vi "Begin.vi"(11 "Image Size":T1=enum."160x120") -> (0 "error out":errorcluster)   [LabVIEW 2011]
doc: "Called before other user functions, this VI is expected to open initial I/O refnums, load in file data, and do all program initialization. Notice that the <B>error out</B> terminal is simply used for data flow. Wiring it to other structures or subVIs ensures that this VI runs first."
uses:
  <vilib>/Rock Robotics/WPI/Camera/WPI_CameraImageSize.ctl
  <vilib>/Rock Robotics/WPI/Joystick/WPI_JoystickDeviceEnum.ctl
  <vilib>/Rock Robotics/WPI/Camera/WPI_CameraWhite Balance Values.ctl
  <vilib>/Rock Robotics/WPI/Camera/WPI_CameraExposure Values.ctl
  <vilib>/Rock Robotics/WPI/Camera/WPI_CameraFrameRate.ctl
  <vilib>/Rock Robotics/SystemInterfaces/DIO/FPGA_DIOPWMChannel.ctl
  <vilib>/Rock Robotics/SystemInterfaces/DIO/FPGA_DIOChannel.ctl
  <vilib>/Rock Robotics/SystemInterfaces/DIO/FPGA_DIORelayChannel.ctl
  <vilib>/Rock Robotics/WPI/RobotDrive/WPI_RobotDriveOpen4MotorWithJaguar.vi
  <vilib>/Rock Robotics/WPI/MotorControl/WPI_MotorControlOpen Jaguar.vi
  <vilib>/Rock Robotics/WPI/Counter/WPI_CounterDigitalInputToDigitalSource.vi
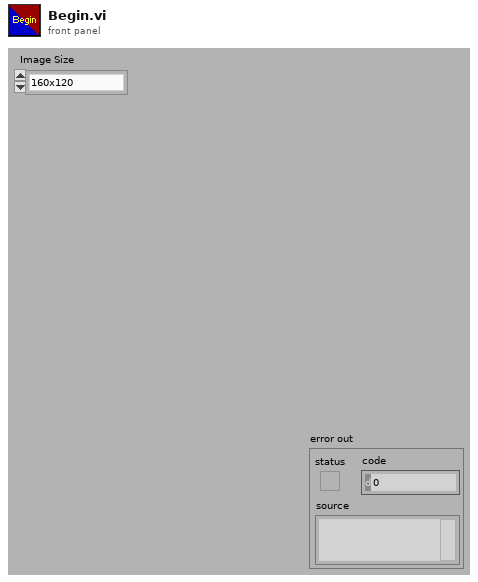
[diagram p1: front panel]
types:
  T1 = typedef "WPI_CameraImageSize.ctl" = enum16{"640x480", "320x240", "160x120"}
  T2 = typedef "FPGA_DIORelayChannel.ctl" = enum8{"Relay 1", "Relay 2", "Relay 3", "Relay 4", "Relay 5", "Relay 6", "Relay 7", "Relay 8", "Invalid"}
  T3 = typedef "FPGA_DIOChannel.ctl" = enum8{"DIO 1", "DIO 2", "DIO 3", "DIO 4", "DIO 5", "DIO 6", "DIO 7", "DIO 8", "DIO 9", "DIO 10", "DIO 11", "DIO 12", "DIO 13", "DIO 14", "Invalid"}
  T4 = typedef "FPGA_DIOPWMChannel.ctl" = enum8{"PWM 1", "PWM 2", "PWM 3", "PWM 4", "PWM 5", "PWM 6", "PWM 7", "PWM 8", "PWM 9", "PWM 10", "Invalid"}
  T5 = typedef "WPI_JoystickDeviceEnum.ctl" = enum16{"USB 1", "USB 2", "USB 3", "USB 4", "Kinect 1", "Kinect 2"}
  T6 = typedef "WPI_CameraFrameRate.ctl" = u32
  T7 = typedef "WPI_CameraExposure Values.ctl" = enum16{"Auto", "Flicker-free 50 Hz", "Flicker-free 60 Hz", "Hold current"}
  T8 = typedef "WPI_CameraWhite Balance Values.ctl" = enum16{"Auto", "Fixed indoor", "Fixed outdoor 1", "Fixed outdoor 2", "Fixed fluorescent 1", "Fixed fluorescent 2", "Hold current"}
  T9 = typedef "WPI_DigitalInputDevRef.ctl" = cluster{"DevStatus":errorcluster, "DIO Channel":T3, "Digital Module":T10}
  T10 = typedef "FPGA_TypedefDigitalModule.ctl" = enum16{"Digital Module 1", "Digital Module 2"}
  T11 = typedef "FPGA_CounterEncoderSourceConvertionLVSourceType.ctl" = cluster{"DevStatus":errorcluster, "AnalogTriggerMode?":bool, "DigitalMode":cluster{"Digital Module":T10, "DIO Channel":T12}, "AnalogTriggerMode":cluster{"AnalogTriggerIndex":T13, "OutputType":T14}}
  T12 = typedef "FPGA_DIODigitalSourceChannel.ctl" = enum8{"DIO 1", "DIO 2", "DIO 3", "DIO 4", "DIO 5", "DIO 6", "DIO 7", "DIO 8", "DIO 9", "DIO 10", "DIO 11", "DIO 12", "DIO 13", "DIO 14", "Disabled"}
  T13 = typedef "FPGA_AnalogTriggerIndex.ctl" = enum8{"Trig 0", "Trig 1", "Trig 2", "Trig 3", "Trig 4", "Trig 5", "Trig 6", "Trig 7", "Invalid"}
  T14 = typedef "FPGA_AnalogTriggerOutType.ctl" = enum16{"InWindow", "TriggerState", "Rising", "Falling"}
  T15 = typedef "WPI_EncoderDevRef.ctl" = cluster{"DevStatus":errorcluster, "EncoderIndex":T16, "CounterIndex":T17, "DistancePerCount":dbl, "Decoding Type":T18}
  T16 = typedef "FPGA_EncoderIdx.ctl" = enum8{"Enc 0", "Enc 1", "Enc 2", "Enc 3", "Invalid"}
  T17 = typedef "FPGA_CounterCtrSystemIndex.ctl" = enum8{"Ctr 0", "Ctr 1", "Ctr 2", "Ctr 3", "Ctr 4", "Ctr 5", "Ctr 6", "Ctr 7", "Invalid"}
  T18 = typedef "WPI_EncoderType.ctl" = enum16{"1x", "2x", "4x"}
  T19 = typedef "WPI_JoystickDevRef.ctl" = cluster{"Device":T5}
  T20 = typedef "WPI_MotorControlDeviceRef.ctl" = cluster{"DeviceStatus":errorcluster, "Type":enum16{"PWM", "CAN"}, "PWM":cluster{"Digital Module":T10, "PWM Channel":T4, "DeadBand":T21}, "CAN":cluster{"Device Number":u8, "Control Mode":T22, "Semaphore":T23, "Max Vout":dbl}, "Invert":bool, "TransformRef":T24, "InvTransformRef":T24}
  T21 = typedef "WPI_PWMDeadband.ctl" = cluster{"Name":string, "maxPositivePwm":i32, "minPositivePwm":i32, "centerPwm":i32, "maxNegativePwm":i32, "minNegativePwm":i32, "angularRange":u16}
  T22 = typedef "WPI_CANJaguar_ControlMode.ctl" = enum8{"Percent VBus", "Current", "Speed", "Position", "Voltage"}
  T23 = typedef "Semaphore RefNum" = refnum<k1>
  T24 = typedef "WPI_PWMTransform_ConPane.ctl" = refnum<vi>
  T25 = typedef "WPI_RobotDriveDevRef.ctl" = cluster{"DevStatus":errorcluster, "Motors[]":T20[], "Square Inputs":bool, "Max Output":dbl, "Isochronous":bool}
  T26 = typedef "WPI_CameraDevRef.ctl" = cluster{"Camera Address":string, "CameraStatus":errorcluster, "Acquire Image Notifier":refnum<notifier>}
  T27 = typedef "WPI_RelayDevRef.ctl" = cluster{"DevStatus":errorcluster, "Relay Channel":T2, "Digital Module":T10, "Relay Direction":T28}
  T28 = typedef "WPI_RelayDirection.ctl" = enum16{"Both directions", "Forward only", "Reverse only"}
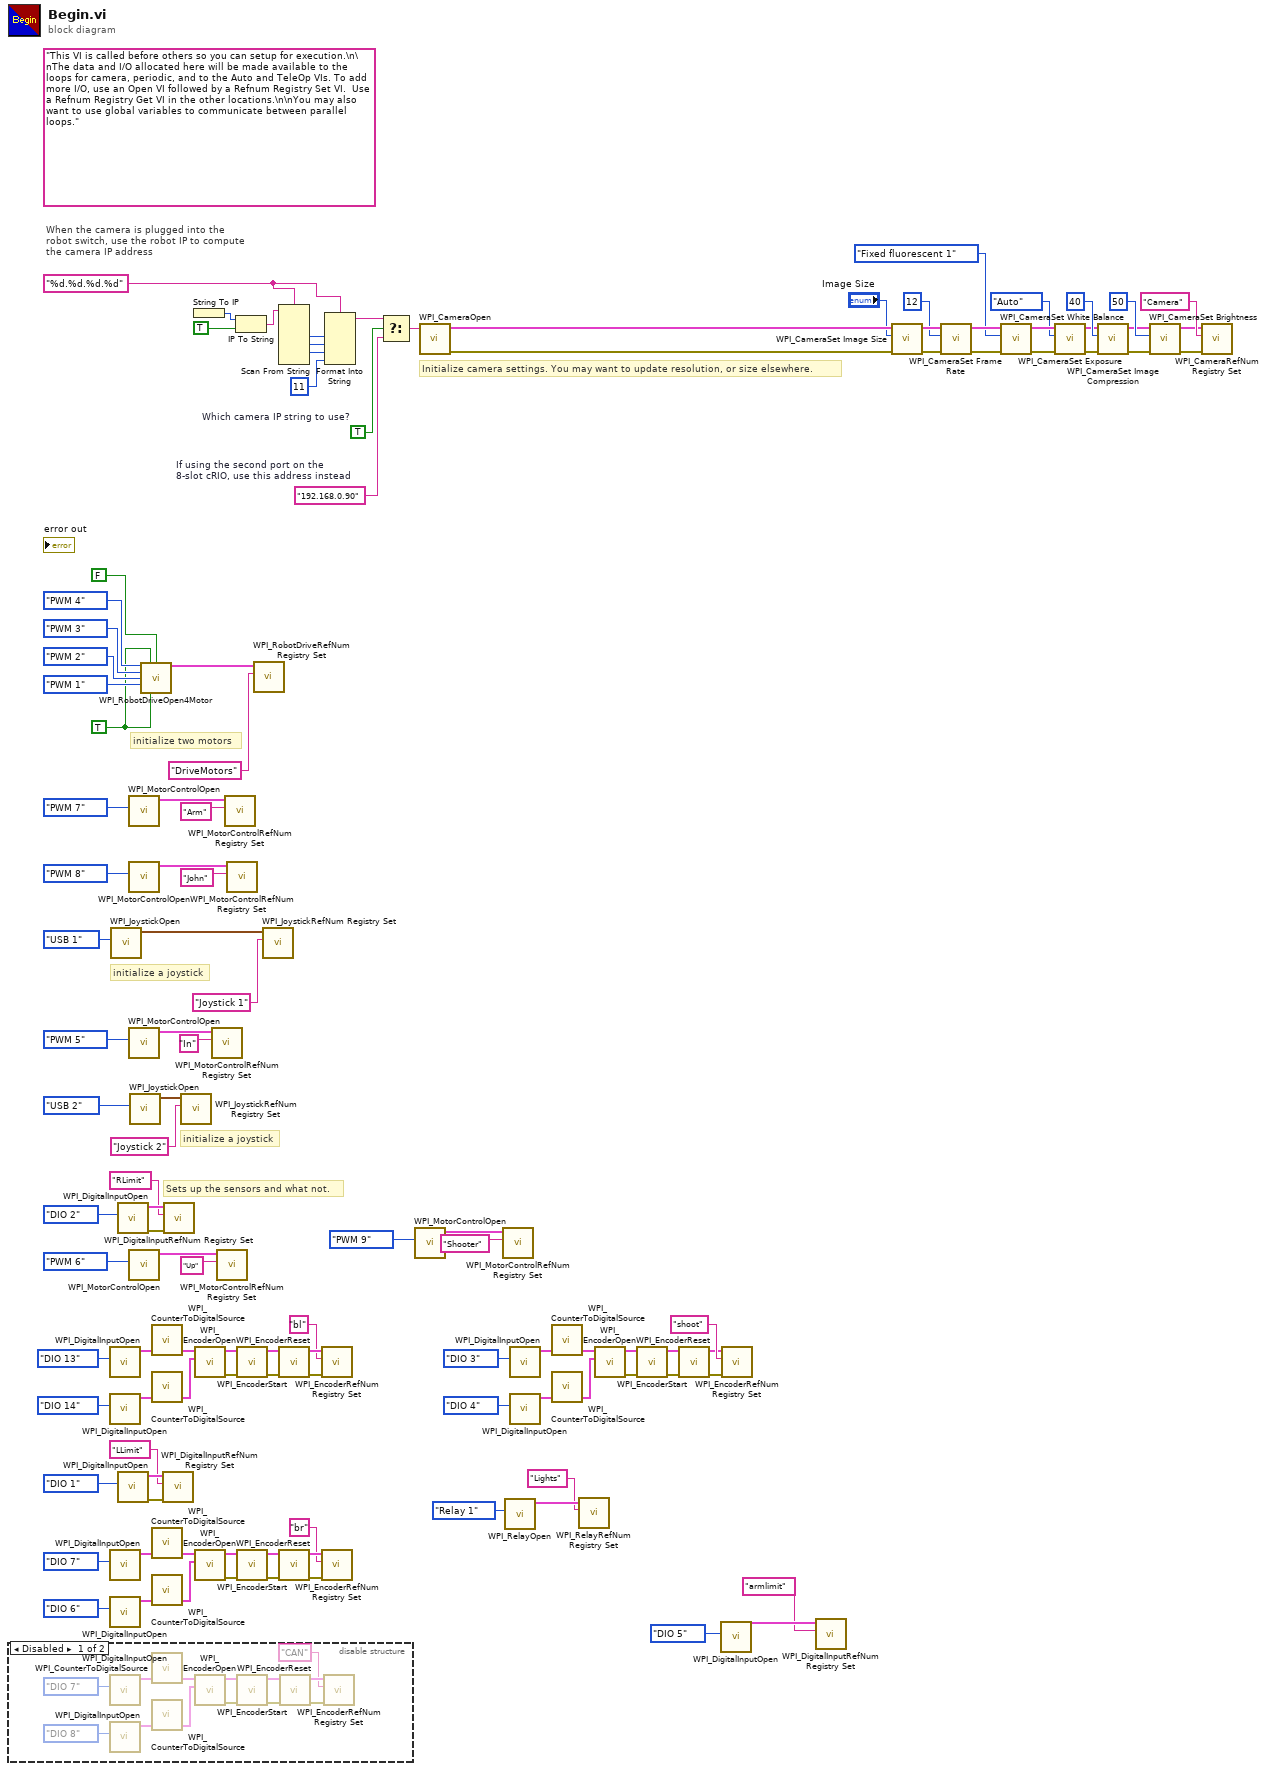
[diagram p0: block diagram]
diagram:
  w49 = TRUE ("Rear Left Motor Inverted")
  w79 = TRUE  # Which camera IP string to use?
  w83 = "%d.%d.%d.%d" ("format string")
  (unwired) "This VI is called before others so you can setup for execution.\n\nThe data and I/O allocated here will be made available to the loops for camera, periodic, and to the Auto and TeleOp VIs. To add more I/O, use an Open VI followed by a Refnum Registry Set VI.  Use a Refnum Registry Get VI in the other locations.\n\nYou may also want to use global variables to communicate between parallel loops."
  w80 = "192.168.0.90"  # If using the second port on the 8-slot cRIO, use this address instead
  # "Sets up the sensors and what not."
  # "initialize a joystick"
  # "When the camera is plugged into the\nrobot switch, use the robot IP to compute\nthe camera IP address"
  # "initialize a joystick"
  # "initialize two motors"
  # "Initialize camera settings. You may want to update resolution, or size elsewhere."
  n1 = disable-structure shown="Disabled" {
    frame Disabled {
      n2 = call <vilib>:"WPI_DigitalInputOpen.vi"("DIO Channel"=FPGA_DIOChannel."DIO 7") -> ("DigitalInputDevRef"=w126:T9)  [unwired: 9 in, 1 out]
      n3 = call <vilib>:"WPI_DigitalInputOpen.vi"("DIO Channel"=FPGA_DIOChannel."DIO 8") -> ("DigitalInputDevRef"=w125:T9)  [unwired: 9 in, 1 out]
      n4 = call-poly <vilib>:"WPI_CounterToDigitalSource.vi"("DigitalInputDevRef"=w126) -> ("Digital Source"=w128:T11)  [unwired: 6 in]
      n5 = call-poly <vilib>:"WPI_CounterToDigitalSource.vi"("DigitalInputDevRef"=w125) -> ("Digital Source"=w127:T11)  [unwired: 6 in]
      n6 = call <vilib>:"WPI_EncoderOpen.vi"("BSource"=w127, "ASource"=w128) -> ("error out"=w122:errorcluster, "EncoderDevRef"=w121:T15)  [unwired: 8 in]
      n7 = call <vilib>:"WPI_EncoderStart.vi"("error in (no error)"=w122, "EncoderDevRef"=w121) -> ("error out"=w120:errorcluster, "EncoderDevRef"=w119:T15)  [unwired: 8 in]
      n8 = call <vilib>:"WPI_EncoderReset.vi"("error in (no error)"=w120, "EncoderDevRef"=w119) -> ("error out"=w118:errorcluster, "EncoderDevRef"=w117:T15)  [unwired: 8 in]
      n9 = call <vilib>:"WPI_EncoderRefNum Registry Set.vi"("error in (no error)"=w118, "refnum name"="CAN", "EncoderDevRef"=w117) -> ()  [unwired: 7 in, 2 out]
    }
    frame Enabled {
    }
  }
  n10 = call <vilib>:"WPI_DigitalInputOpen.vi"("DIO Channel"=FPGA_DIOChannel."DIO 13") -> ("DigitalInputDevRef"=w48:T9)  [unwired: 9 in, 1 out]
  n11 = call <vilib>:"WPI_DigitalInputOpen.vi"("DIO Channel"=FPGA_DIOChannel."DIO 14") -> ("DigitalInputDevRef"=w43:T9)  [unwired: 9 in, 1 out]
  n12 = call <vilib>:"WPI_DigitalInputOpen.vi"("DIO Channel"=FPGA_DIOChannel."DIO 7") -> ("DigitalInputDevRef"=w42:T9)  [unwired: 9 in, 1 out]
  n13 = call <vilib>:"WPI_DigitalInputOpen.vi"("DIO Channel"=FPGA_DIOChannel."DIO 6") -> ("DigitalInputDevRef"=w41:T9)  [unwired: 9 in, 1 out]
  n14 = call <vilib>:"WPI_JoystickOpen.vi"("JoystickDevice"=WPI_JoystickDeviceEnum."USB 1") -> ("JoystickDevRef"=w113:T19)  [unwired: 10 out]
  n15 = call <vilib>:"WPI_DigitalInputOpen.vi"("DIO Channel"=FPGA_DIOChannel."DIO 2") -> ("error out"=w57:errorcluster, "DigitalInputDevRef"=w56:T9)  [unwired: 9 in]
  n16 = call <vilib>:"WPI_DigitalInputOpen.vi"("DIO Channel"=FPGA_DIOChannel."DIO 1") -> ("error out"=w53:errorcluster, "DigitalInputDevRef"=w52:T9)  [unwired: 9 in]
  n17 = call-poly <vilib>:"WPI_MotorControlOpen.vi"("PWM Channel"=FPGA_DIOPWMChannel."PWM 7") -> ("MotorControlDeviceRef"=w72:T20)  [unwired: 9 in, 1 out]
  n18 = call-poly <vilib>:"WPI_MotorControlOpen.vi"("PWM Channel"=FPGA_DIOPWMChannel."PWM 8") -> ("MotorControlDeviceRef"=w66:T20)  [unwired: 9 in, 1 out]
  n19 = call-poly <vilib>:"WPI_MotorControlOpen.vi"("PWM Channel"=FPGA_DIOPWMChannel."PWM 5") -> ("MotorControlDeviceRef"=w63:T20)  [unwired: 9 in, 1 out]
  n20 = call-poly <vilib>:"WPI_MotorControlOpen.vi"("PWM Channel"=FPGA_DIOPWMChannel."PWM 6") -> ("MotorControlDeviceRef"=w60:T20)  [unwired: 9 in, 1 out]
  n21 = call <vilib>:"WPI_JoystickOpen.vi"("JoystickDevice"=WPI_JoystickDeviceEnum."USB 2") -> ("JoystickDevRef"=w71:T19)  [unwired: 10 out]
  n22 = call-poly <vilib>:"WPI_RobotDriveOpen4Motor.vi"("Rear Left Motor"=FPGA_DIOPWMChannel."PWM 4", "Rear Left Motor Inverted"=w49, "Rear Right Motor Inverted"=FALSE, "Rear Right Motor"=FPGA_DIOPWMChannel."PWM 3", "Front Left Motor"=FPGA_DIOPWMChannel."PWM 2", "Front Right Motor"=FPGA_DIOPWMChannel."PWM 1", "Front Left Motor Inverted"=w49) -> ("RobotDriveDevRef"=w78:T25)  [unwired: 7 in, 1 out]
  n23 = call-poly <vilib>:"WPI_CounterToDigitalSource.vi"("DigitalInputDevRef"=w48) -> ("Digital Source"=w47:T11)  [unwired: 6 in]
  n24 = call-poly <vilib>:"WPI_CounterToDigitalSource.vi"("DigitalInputDevRef"=w43) -> ("Digital Source"=w44:T11)  [unwired: 6 in]
  n25 = call-poly <vilib>:"WPI_CounterToDigitalSource.vi"("DigitalInputDevRef"=w42) -> ("Digital Source"=w46:T11)  [unwired: 6 in]
  n26 = call-poly <vilib>:"WPI_CounterToDigitalSource.vi"("DigitalInputDevRef"=w41) -> ("Digital Source"=w45:T11)  [unwired: 6 in]
  n27 = call <vilib>:"WPI_DigitalInputRefNum Registry Set.vi"("error in (no error)"=w53, "refnum name"="LLimit", "DigitalInputDevRef"=w52) -> ()  [unwired: 7 in, 2 out]
  n28 = call <vilib>:"WPI_DigitalInputRefNum Registry Set.vi"("error in (no error)"=w57, "refnum name"="RLimit", "DigitalInputDevRef"=w56) -> ()  [unwired: 7 in, 2 out]
  n29 = call <vilib>:"WPI_JoystickRefNum Registry Set.vi"("refnum name"="Joystick 2", "JoystickDevRef"=w71) -> ()  [unwired: 1 in, 9 out]
  n30 = String To IP() -> (0:w90:u32)  [unwired: 1 in]
  n31 = call <vilib>:"WPI_EncoderOpen.vi"("BSource"=w44, "ASource"=w47) -> ("error out"=w31:errorcluster, "EncoderDevRef"=w32:T15)  [unwired: 8 in]
  n32 = call <vilib>:"WPI_EncoderOpen.vi"("BSource"=w45, "ASource"=w46) -> ("error out"=w34:errorcluster, "EncoderDevRef"=w33:T15)  [unwired: 8 in]
  n33 = call <vilib>:"WPI_MotorControlRefNum Registry Set.vi"("refnum name"="In", "MotorControlDevRef"=w63) -> ()  [unwired: 8 in, 2 out]
  n34 = call <vilib>:"WPI_MotorControlRefNum Registry Set.vi"("refnum name"="Up", "MotorControlDevRef"=w60) -> ()  [unwired: 8 in, 2 out]
  n35 = call <vilib>:"WPI_MotorControlRefNum Registry Set.vi"("refnum name"="Arm", "MotorControlDevRef"=w72) -> ()  [unwired: 8 in, 2 out]
  n36 = call <vilib>:"WPI_MotorControlRefNum Registry Set.vi"("refnum name"="John", "MotorControlDevRef"=w66) -> ()  [unwired: 8 in, 2 out]
  n37 = IP To String(1:TRUE ("dot notation? (F)"), 2:w90) -> (0:w88:string)
  n38 = call <vilib>:"WPI_EncoderStart.vi"("error in (no error)"=w31, "EncoderDevRef"=w32) -> ("error out"=w36:errorcluster, "EncoderDevRef"=w35:T15)  [unwired: 8 in]
  n39 = call <vilib>:"WPI_EncoderStart.vi"("error in (no error)"=w34, "EncoderDevRef"=w33) -> ("error out"=w30:errorcluster, "EncoderDevRef"=w29:T15)  [unwired: 8 in]
  n40 = call <vilib>:"WPI_RobotDriveRefNum Registry Set.vi"("refnum name"="DriveMotors", "RobotDriveDevRef"=w78) -> ()  [unwired: 1 in, 9 out]
  n41 = call <vilib>:"WPI_JoystickRefNum Registry Set.vi"("refnum name"="Joystick 1", "JoystickDevRef"=w113) -> ()  [unwired: 1 in, 9 out]
  n42 = Scan From String(format string=w83, input string=w88) -> (output 1=w87:i32, output 2=w86:i32, output 3=w85:i32)  [unwired: 7 in, 3 out]
  n43 = call <vilib>:"WPI_EncoderReset.vi"("error in (no error)"=w36, "EncoderDevRef"=w35) -> ("error out"=w28:errorcluster, "EncoderDevRef"=w27:T15)  [unwired: 8 in]
  n44 = call <vilib>:"WPI_EncoderReset.vi"("error in (no error)"=w30, "EncoderDevRef"=w29) -> ("error out"=w25:errorcluster, "EncoderDevRef"=w26:T15)  [unwired: 8 in]
  n45 = call <vilib>:"WPI_EncoderRefNum Registry Set.vi"("error in (no error)"=w28, "refnum name"="bl", "EncoderDevRef"=w27) -> ()  [unwired: 7 in, 2 out]
  n46 = call <vilib>:"WPI_EncoderRefNum Registry Set.vi"("error in (no error)"=w25, "refnum name"="br", "EncoderDevRef"=w26) -> ()  [unwired: 7 in, 2 out]
  n47 = Format Into String(format string=w83, w87, w86, w85, 11 ("Compression")) -> (resulting string=w81:string)  [unwired: 2 in, 1 out]
  n48 = Select(t=w81, s=w79, f=w80) -> (s? t:f=w82:string)
  n49 = call-poly <vilib>:"WPI_MotorControlOpen.vi"("PWM Channel"=FPGA_DIOPWMChannel."PWM 9") -> ("MotorControlDeviceRef"=w22:T20)  [unwired: 9 in, 1 out]
  n50 = call <vilib>:"WPI_CameraOpen.vi"("Camera Address"=w82) -> ("error out"=w103:errorcluster, "CameraDevRef"=w104:T26)  [unwired: 1 in, 8 out]
  n51 = call <vilib>:"WPI_MotorControlRefNum Registry Set.vi"("refnum name"="Shooter", "MotorControlDevRef"=w22) -> ()  [unwired: 8 in, 2 out]
  n52 = call <vilib>:"WPI_RelayOpen.vi"("Relay Channel"=FPGA_DIORelayChannel."Relay 1") -> ("RelayDevRef"=w2:T27)  [unwired: 9 in, 1 out]
  n53 = call <vilib>:"WPI_DigitalInputOpen.vi"("DIO Channel"=FPGA_DIOChannel."DIO 3") -> ("DigitalInputDevRef"=w4:T9)  [unwired: 9 in, 1 out]
  n54 = call <vilib>:"WPI_DigitalInputOpen.vi"("DIO Channel"=FPGA_DIOChannel."DIO 4") -> ("DigitalInputDevRef"=w7:T9)  [unwired: 9 in, 1 out]
  n55 = call-poly <vilib>:"WPI_CounterToDigitalSource.vi"("DigitalInputDevRef"=w4) -> ("Digital Source"=w5:T11)  [unwired: 6 in]
  n56 = call-poly <vilib>:"WPI_CounterToDigitalSource.vi"("DigitalInputDevRef"=w7) -> ("Digital Source"=w6:T11)  [unwired: 6 in]
  n57 = call <vilib>:"WPI_RelayRefNum Registry Set.vi"("refnum name"="Lights", "RelayDevRef"=w2) -> ()  [unwired: 8 in, 2 out]
  n58 = call <vilib>:"WPI_EncoderOpen.vi"("BSource"=w6, "ASource"=w5) -> ("error out"=w13:errorcluster, "EncoderDevRef"=w12:T15)  [unwired: 8 in]
  n59 = call <vilib>:"WPI_EncoderStart.vi"("error in (no error)"=w13, "EncoderDevRef"=w12) -> ("error out"=w10:errorcluster, "EncoderDevRef"=w11:T15)  [unwired: 8 in]
  n60 = call <vilib>:"WPI_EncoderReset.vi"("error in (no error)"=w10, "EncoderDevRef"=w11) -> ("error out"=w14:errorcluster, "EncoderDevRef"=w15:T15)  [unwired: 8 in]
  n61 = call <vilib>:"WPI_DigitalInputOpen.vi"("DIO Channel"=FPGA_DIOChannel."DIO 5") -> ("DigitalInputDevRef"=w19:T9)  [unwired: 9 in, 1 out]
  n62 = call <vilib>:"WPI_EncoderRefNum Registry Set.vi"("error in (no error)"=w14, "refnum name"="shoot", "EncoderDevRef"=w15) -> ()  [unwired: 7 in, 2 out]
  n63 = call <vilib>:"WPI_DigitalInputRefNum Registry Set.vi"("refnum name"="armlimit", "DigitalInputDevRef"=w19) -> ()  [unwired: 8 in, 2 out]
  n64 = call <vilib>:"WPI_CameraSet Image Size.vi"("error in (no error)"=w103, "Image Size"="Image Size", "CameraDevRef"=w104) -> ("error out"=w102:errorcluster, "CameraDevRef Out"=w105:T26)  [unwired: 7 out]
  n65 = call <vilib>:"WPI_CameraSet Frame Rate.vi"("error in (no error)"=w102, "Frame Rate (fps)"=T6 12, "CameraDevRef"=w105) -> ("error out"=w101:errorcluster, "CameraDevRef Out"=w107:T26)  [unwired: 7 out]
  n66 = call <vilib>:"WPI_CameraSet White Balance.vi"("error in (no error)"=w101, "White Balance"=WPI_CameraWhite_Balance_Values."Fixed fluorescent 1", "CameraDevRef"=w107) -> ("error out"=w100:errorcluster, "CameraDevRef Out"=w106:T26)  [unwired: 7 out]
  n67 = call <vilib>:"WPI_CameraSet Exposure.vi"("error in (no error)"=w100, "Exposure"=WPI_CameraExposure_Values."Auto", "CameraDevRef"=w106) -> ("error out"=w99:errorcluster, "CameraDevRef Out"=w109:T26)  [unwired: 7 out]
  n68 = call <vilib>:"WPI_CameraSet Image Compression.vi"("error in (no error)"=w99, "Compression"=40, "CameraDevRef"=w109) -> ("error out"=w98:errorcluster, "CameraDevRef Out"=w108:T26)  [unwired: 7 out]
  n69 = call <vilib>:"WPI_CameraSet Brightness.vi"("error in (no error)"=w98, "Brightness"=50, "CameraDevRef"=w108) -> ("error out"=w96:errorcluster, "CameraDevRef Out"=w97:T26)  [unwired: 7 out]
  n70 = call <vilib>:"WPI_CameraRefNum Registry Set.vi"("error in (no error)"=w96, "refnum name"="Camera", "CameraDevRef"=w97) -> ()  [unwired: 9 out]
